vi "synnax channel retrieve keys Array.vi"(0 "client":u64, 5 "names":string[](array[numeric]), 11 "error in (no error)":errorcluster) -> (4 "client out":u64, 6 "keys":u32[](array[numeric]), 15 "error out":errorcluster)   [LabVIEW 2026, in "synnax_clib.lvlib"]
doc: "SYNNAX_EXPORT int32_t synnax_channel_retrieve_keys(\n SynnaxClient client,\n const char **names,\n uint64_t name_count,\n uint32_t *out_keys,\n SynnaxError err\n);"
uses:
  synnax_clib.lvlib
  synnax_clib.dll
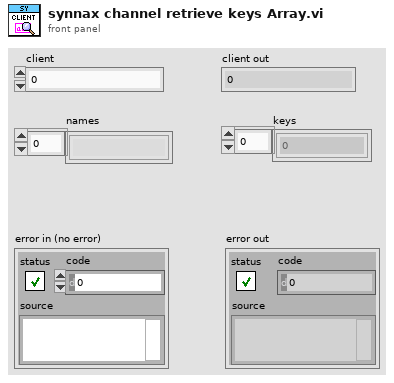
[diagram p1: front panel]
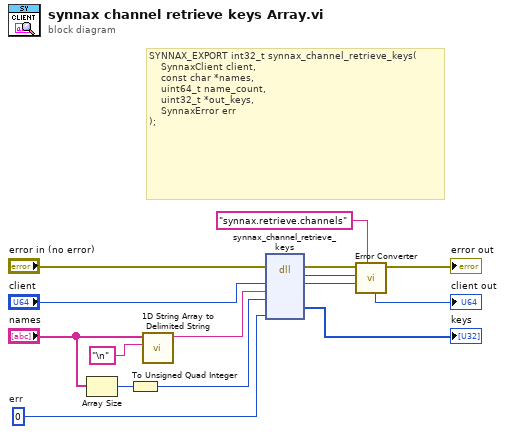
[diagram p0: block diagram]
diagram:
  w3 = u64 0  # err
  # "SYNNAX_EXPORT int32_t synnax_channel_retrieve_keys(\n    SynnaxClient client,\n    const char *names,\n    uint64_t name_count,\n    uint32_t *out_keys,\n    SynnaxError err\n);"
  n1 = Array Size(array="names") -> (size(s)=w9:i32)
  n2 = To Unsigned Quad Integer(1:w9) -> (0:w8:u64)
  n3 = call <vilib>:"1D String Array to Delimited String.vi"("delimiter"="\n", "string array"="names") -> ("delimited string"=w2:string)  [unwired: 9 in]
  n4 = dll-call lib="C/synnax/client/labview/synnax_clib.*" fn="synnax_channel_retrieve_keys"(error in="error in (no error)", "client"="client", "names"=w2, "name_count"=w8, "err"=w3) -> (error out=w5:errorcluster, "return type"=w7:i32, "client"=→"client out":u64, "out_keys"=→"keys":u32[])  [unwired: 6 in, 1 out]
  n5 = call "Error Converter.vi"("source"="synnax.retrieve.channels", "error code"=w7, "error in (no error)"=w5) -> ("error out"=→"error out":errorcluster)  [unwired: 8 in]
